vi "QueueMidi.vi"() -> ()   [LabVIEW 2014]
panel:
  out "Stopping":bool
  out "Read Data":i32
  in  "stop":bool
  out "error out":errorcluster
  in  "Queue Name":string="Midi In"
  in  "error in":errorcluster
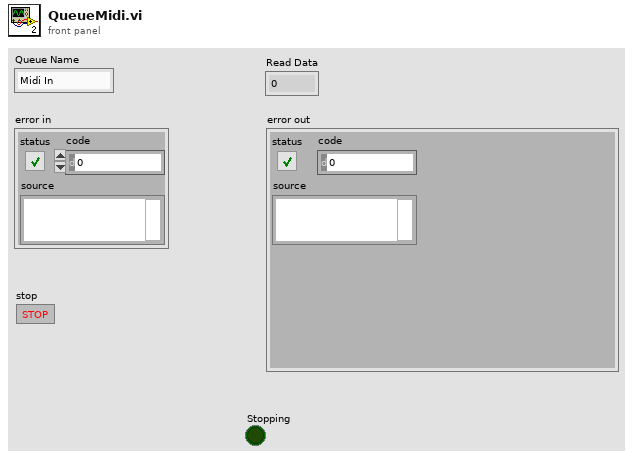
[diagram p1: front panel]
types:
  T1 = cluster{"Invert Polarity?":bool, "baud rate (312500)":u32, "data bits (8)":u16, "parity (0:none)":u16, "stop bits (10: 1 bit)":u16}
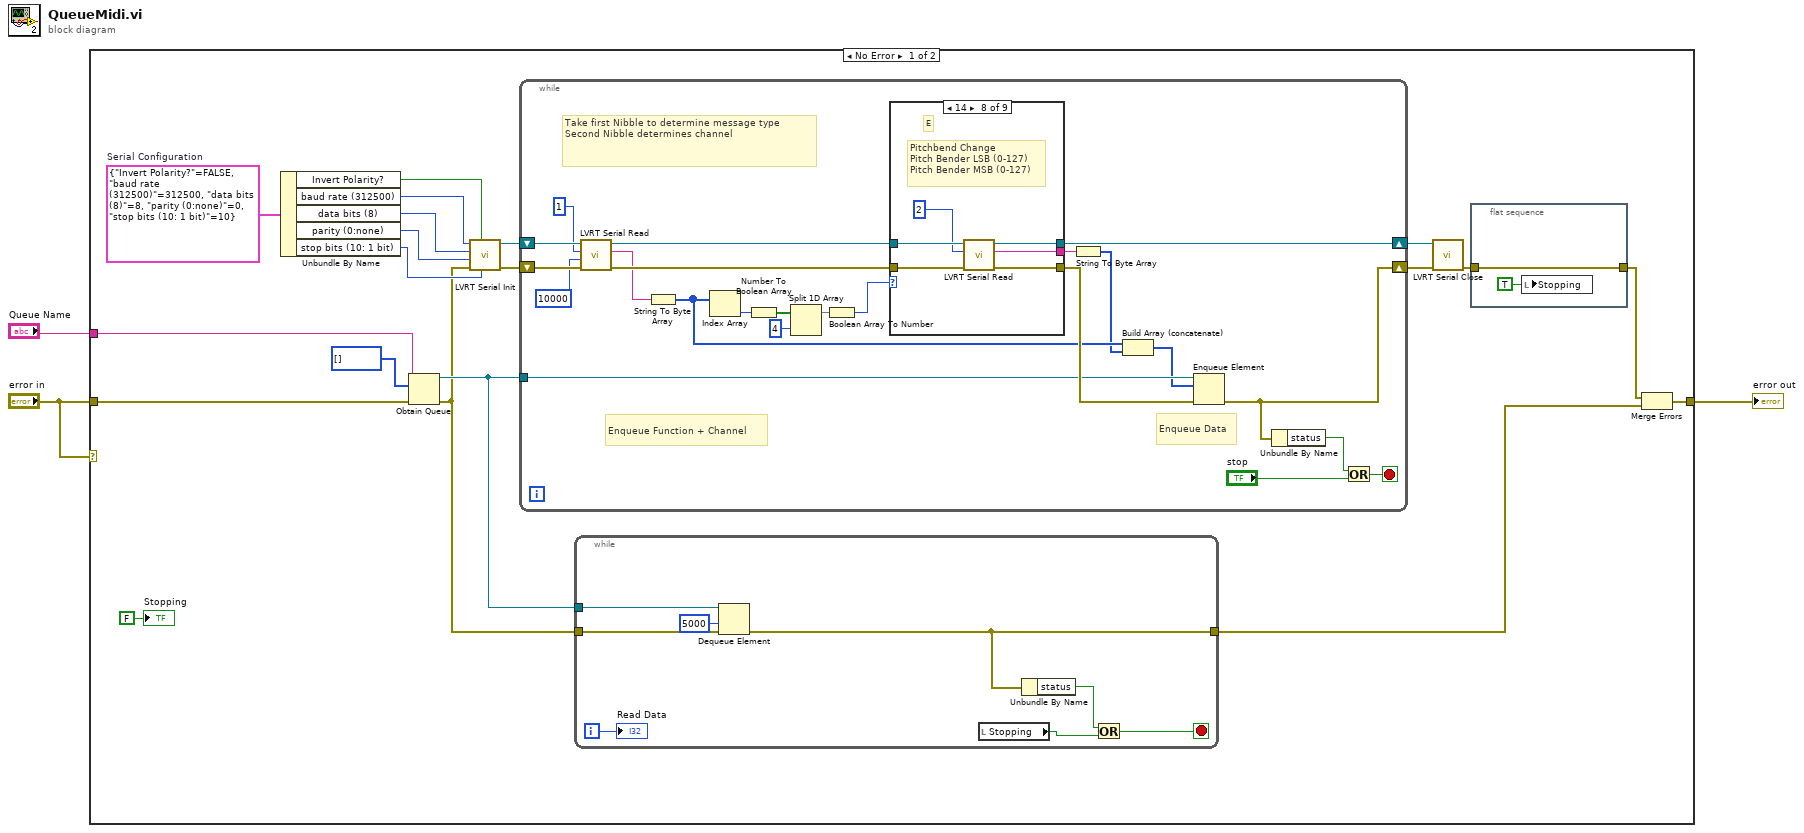
[diagram p0: block diagram]
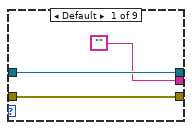
[diagram p2: hidden frame]
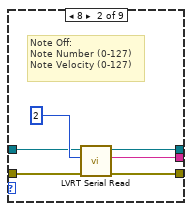
[diagram p3: hidden frame]
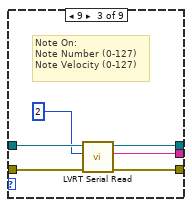
[diagram p4: hidden frame]
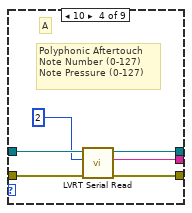
[diagram p5: hidden frame]
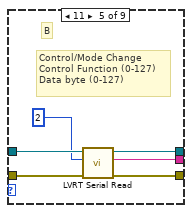
[diagram p6: hidden frame]
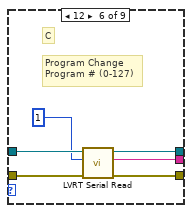
[diagram p7: hidden frame]
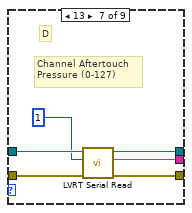
[diagram p8: hidden frame]
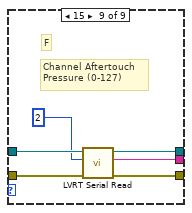
[diagram p9: hidden frame]
diagram:
  n1 = case shown="No Error" "error in" {
    tunnel: "error in" -> [w23 w108]
    tunnel: [w8 w108] -> w1
    tunnel: "Queue Name" -> [w22 _]
    frame No Error {
      w18 = T1 {"Invert Polarity?"=FALSE, "baud rate (312500)"=312500, "data bits (8)"=8, "parity (0:none)"=0, "stop bits (10: 1 bit)"=10}  # Serial Configuration
      n2 = Unbundle By Name(w18) -> ("Invert Polarity?"=w17:bool, "baud rate (312500)"=w16:u32, "data bits (8)"=w15:u16, "parity (0:none)"=w14:u16, "stop bits (10: 1 bit)"=w13:u16)
      n3 = Obtain Queue(name (unnamed)=w22, element data type=u8[] [] ("unsigned byte array"), error in (no error)=w23) -> (queue out=w10:refnum<queue>, error out=w9:errorcluster)  [unwired: 2 in, 1 out]
      n4 = call "LVRT Serial Init.vi"("stop bits (10: 1 bit)"=w13, "Invert Polarity?"=w17, "error in (no error)"=w9, "parity (0:none)"=w14, "data bits (8)"=w15, "baud rate (9600)"=w16) -> ("error out"=w20:errorcluster, "FPGA Main Reference Out"=w19:refnum<k20>)  [unwired: 4 in]
      n5 = while {
        shift-right: [w56] -> w11
        shift-left: w19 -> [w44]
        tunnel: w10 -> [w49]
        shift-right: [w35] -> w12
        shift-left: w20 -> [w43]
        stop <- w36 stop-if-true
        # "Enqueue Data"
        # "Enqueue Function + Channel"
        # "Take first Nibble to determine message type\nSecond Nibble determines channel"
        n6 = call "LVRT Serial Read.vi"("error in (no error)"=w43, "Timeout (ms) (-1: no timeout)"=10000, "Bytes to Read"=u32 1 ("byte count"), "FPGA Main Ref"=w44) -> ("error out"=w42:errorcluster, "String"=w41:string, "FPGA Main Ref Out"=w39:refnum<k20>)  [unwired: 1 in, 4 out]
        n7 = String To Byte Array(string=w41) -> (unsigned byte array=w47:u8[])
        n8 = Index Array(array=w47) -> (element=w55:u8)  [unwired: 1 in]
        n9 = Number To Boolean Array(number=w55) -> (Boolean array=w54:bool[])
        n10 = Split 1D Array(array=w54, index=4) -> (first subarray=w52:bool[])  [unwired: 1 out]
        n11 = Boolean Array To Number(Boolean array=w52) -> (number=w51:u32)
        n12 = case shown="14" w51 {
          tunnel: w39 -> [w59 w64 w71 w77 w83 w89 w95 w101 w107]
          tunnel: [w59 w60 w67 w73 w79 w85 w91 w97 w103] -> w56
          tunnel: ["" w61 w68 w74 w80 w86 w92 w98 w104] -> w48
          tunnel: [w57 w62 w69 w75 w81 w87 w93 w99 w105] -> w50
          tunnel: w42 -> [w57 w63 w70 w76 w82 w88 w94 w100 w106]
          frame Default {
          }
          frame 8 {
            # "Note Off: \nNote Number (0-127)\nNote Velocity (0-127)"
            n13 = call "LVRT Serial Read.vi"("error in (no error)"=w63, "Bytes to Read"=u32 2 ("byte count"), "FPGA Main Ref"=w64) -> ("error out"=w62:errorcluster, "String"=w61:string, "FPGA Main Ref Out"=w60:refnum<k20>)  [unwired: 2 in, 4 out]
          }
          frame 9 {
            # "Note On: \nNote Number (0-127)\nNote Velocity (0-127)"
            n14 = call "LVRT Serial Read.vi"("error in (no error)"=w70, "Bytes to Read"=u32 2 ("byte count"), "FPGA Main Ref"=w71) -> ("error out"=w69:errorcluster, "String"=w68:string, "FPGA Main Ref Out"=w67:refnum<k20>)  [unwired: 2 in, 4 out]
          }
          frame 10 {
            # "A"
            # "Polyphonic Aftertouch\nNote Number (0-127)\nNote Pressure (0-127)"
            n15 = call "LVRT Serial Read.vi"("error in (no error)"=w76, "Bytes to Read"=u32 2 ("byte count"), "FPGA Main Ref"=w77) -> ("error out"=w75:errorcluster, "String"=w74:string, "FPGA Main Ref Out"=w73:refnum<k20>)  [unwired: 2 in, 4 out]
          }
          frame 11 {
            # "B"
            # "Control/Mode Change\nControl Function (0-127)\nData byte (0-127)"
            n16 = call "LVRT Serial Read.vi"("error in (no error)"=w82, "Bytes to Read"=u32 2 ("byte count"), "FPGA Main Ref"=w83) -> ("error out"=w81:errorcluster, "String"=w80:string, "FPGA Main Ref Out"=w79:refnum<k20>)  [unwired: 2 in, 4 out]
          }
          frame 12 {
            # "C"
            # "Program Change\nProgram # (0-127)"
            n17 = call "LVRT Serial Read.vi"("error in (no error)"=w88, "Bytes to Read"=u32 1 ("byte count"), "FPGA Main Ref"=w89) -> ("error out"=w87:errorcluster, "String"=w86:string, "FPGA Main Ref Out"=w85:refnum<k20>)  [unwired: 2 in, 4 out]
          }
          frame 13 {
            # "Channel Aftertouch\nPressure (0-127)"
            # "D"
            n18 = call "LVRT Serial Read.vi"("error in (no error)"=w94, "Bytes to Read"=u32 1 ("byte count"), "FPGA Main Ref"=w95) -> ("error out"=w93:errorcluster, "String"=w92:string, "FPGA Main Ref Out"=w91:refnum<k20>)  [unwired: 2 in, 4 out]
          }
          frame 14 {
            # "E"
            # "Pitchbend Change\nPitch Bender LSB (0-127)\nPitch Bender MSB (0-127)"
            n19 = call "LVRT Serial Read.vi"("error in (no error)"=w100, "Bytes to Read"=u32 2 ("byte count"), "FPGA Main Ref"=w101) -> ("error out"=w99:errorcluster, "String"=w98:string, "FPGA Main Ref Out"=w97:refnum<k20>)  [unwired: 2 in, 4 out]
          }
          frame 15 {
            # "F"
            # "Channel Aftertouch\nPressure (0-127)"
            n20 = call "LVRT Serial Read.vi"("error in (no error)"=w106, "Bytes to Read"=u32 2 ("byte count"), "FPGA Main Ref"=w107) -> ("error out"=w105:errorcluster, "String"=w104:string, "FPGA Main Ref Out"=w103:refnum<k20>)  [unwired: 2 in, 4 out]
          }
        }
        n21 = String To Byte Array(string=w48) -> (unsigned byte array=w46:u8[])
        n22 = Build Array (concatenate)(w47, w46) -> (w45:u8[])
        n23 = Enqueue Element(queue=w49, element=w45, error in (no error)=w50) -> (error out=w35:errorcluster)  [unwired: 1 in, 2 out]
        n24 = Unbundle By Name(w35) -> ("status"=w38:bool)
        n25 = Or(x=w38, y="stop") -> (x .or. y?=w36:bool)
      }
      n26 = while {
        tunnel: w10 -> [w33]
        tunnel: w9 -> [w32]
        tunnel: [w29] -> w7
        i -> [w28]
        stop <- w30 stop-if-true
        n27 = Dequeue Element(queue=w33, timeout in ms (-1)=5000, error in (no error)=w32) -> (error out=w29:errorcluster)  [unwired: 3 out]
        n28 = local read "Stopping"() -> (w27:bool)
        n29 = Unbundle By Name(w29) -> ("status"=w31:bool)
        n30 = Or(x=w31, y=w27) -> (x .or. y?=w30:bool)
        "Read Data" <- w28
      }
      n31 = call "LVRT Serial Close.vi"("error out"=w12, "FPGA Main Ref"=w11) -> ("error out"=w6:errorcluster)  [unwired: 9 in]
      n32 = flat-sequence {
        tunnel: w6 -> [w25]
        tunnel: [w25] -> w5
        frame #0 {
          n33 = local write "Stopping"(TRUE ("Stopping")) -> ()
        }
      }
      n34 = Merge Errors(w5, w7) -> (w8:errorcluster)
      "Stopping" <- FALSE ("Stopping")
    }
    frame Error {
    }
  }
  "error out" <- w1
